vi "Receive Panel Close Event.vi"(8 "error in (no error)":errorcluster, 10 "PanelCloseMsg":refnum<class "PanelCloseMsg.lvclass">, 11 "TwoButtonDialogBox in":refnum<class "TwoButtonDialogBox.lvclass">) -> (0 "error out":errorcluster, 3 "TwoButtonDialogBox out":refnum<class "TwoButtonDialogBox.lvclass">)   [LabVIEW 2017, in "TwoButtonDialogBox.lvlib" / "TwoButtonDialogBox.lvclass"]
doc: "<License>\nCopyright © 2017 Composed Systems, LLC | All rights reserved\nwww.composed.io\n\nAuthor: Ethan Stern <ethan.stern@composed.io>\n\nThis software is provided \"AS IS\" WITHOUT WARRANTIES, either express or implied, AND IS FOR EDUCATIONAL PURPOSES ONLY.\n</License>"
uses:
  TwoButtonDialogBox.lvclass
  C:/Program Files (x86)/National Instruments/LabVIEW 2017/vi.lib/ActorFramework/Actor/Actor.lvclass
  Framework/ActorEvents/IEventAggregator Messages/PanelCloseMsg/PanelCloseMsg.lvclass
  <vilib>/ActorFramework/Actor/Actor.lvclass/Actor.ctl
  <vilib>/ActorFramework/Message Enqueuer/Message Enqueuer.lvclass/Message Enqueuer.ctl
  TwoButtonDialogBox.lvclass/TwoButtonDialogBox.ctl
  <vilib>/ActorFramework/Message Enqueuer/Init from Existing Queue.vi
  <vilib>/ActorFramework/Message Enqueuer/Enqueue.vi
  <vilib>/ActorFramework/Stop Msg/Stop Msg.lvclass
  C:/Program Files (x86)/National Instruments/LabVIEW 2017/vi.lib/ActorFramework/Message/Message.lvclass
  <vilib>/ActorFramework/Message Priority Queue/Priority Enqueue.vi
  <vilib>/ActorFramework/Message Enqueuer/Message Enqueuer.lvclass
  Framework/IDialogBox/IDialogBox Messages/Dialog Return Msg/Dialog Return Msg.lvclass
  <vilib>/ActorFramework/Actor/Actor.lvclass
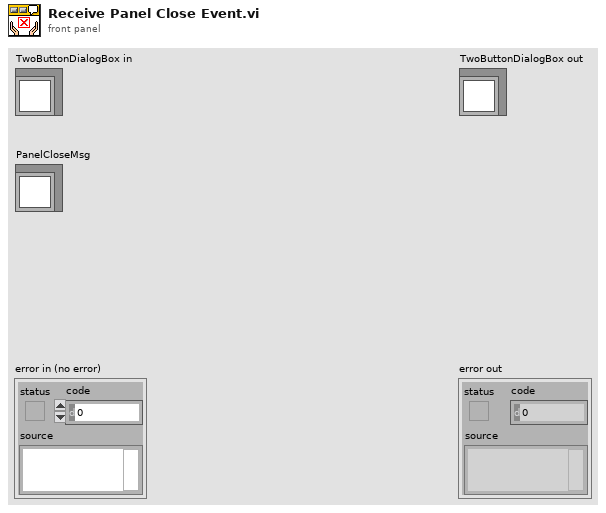
[diagram p1: front panel]
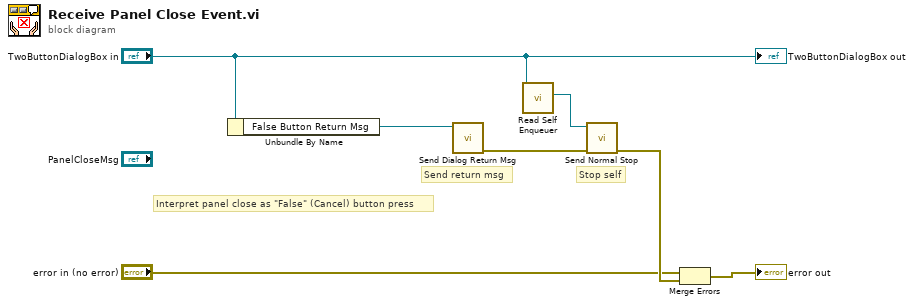
[diagram p0: block diagram]
diagram:
  # "Interpret panel close as \"False\" (Cancel) button press"
  # "Stop self"
  # "Send return msg"
  n1 = Unbundle By Name("TwoButtonDialogBox in") -> ("False Button Return Msg"=w1:refnum<class "Dialog Return Msg.lvclass">)
  n2 = call "Send Dialog Return Msg.vi"("Dialog Return Msg"=w1) -> ("error out"=w5:errorcluster)  [unwired: 10 in]
  n3 = call <vilib>:"Read Self Enqueuer.vi"("Actor"="TwoButtonDialogBox in") -> ("Self Enqueuer"=w6:refnum<class "Message Enqueuer.lvclass">)  [unwired: 10 in]
  n4 = call <vilib>:"Send Normal Stop.vi"("error in (no error)"=w5, "Message Enqueuer"=w6) -> ("error out"=w7:errorcluster)  [unwired: 9 in]
  n5 = Merge Errors("error in (no error)", w7) -> (→"error out":errorcluster)
  "TwoButtonDialogBox out" <- "TwoButtonDialogBox in"
